vi "sonar_position_difference.vi"(2 "Obstacles":dbl[][](array[numeric]), 3 "Car.lvclass":refnum<class "Car.lvclass">, 4 "Sonar Readings":dbl[](array[numeric])) -> (0 "Y Difference":dbl, 1 "X Difference":dbl)   [LabVIEW 2015]
uses:
  class/Car.lvclass
  class/SonarSensor.lvclass
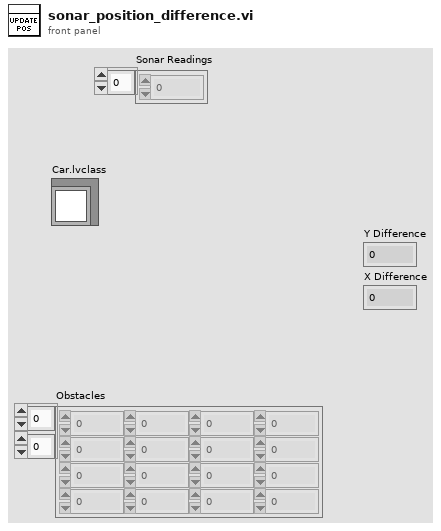
[diagram p1: front panel]
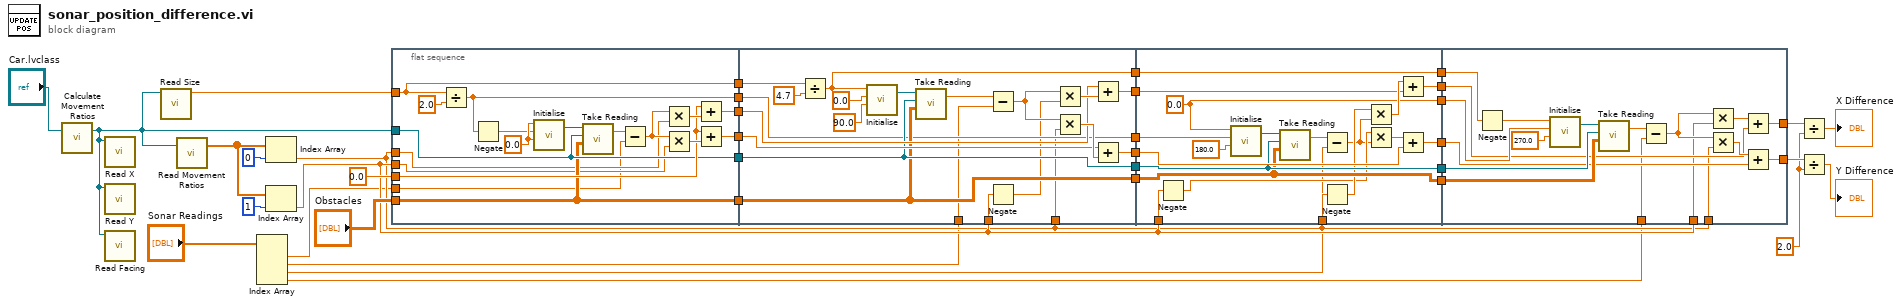
[diagram p0: block diagram]
diagram:
  w11 = 2.0 ("y")
  n1 = call "Calculate Movement Ratios.vi"("Car.lvclass"="Car.lvclass") -> ("Car.lvclass 2"=w1:refnum<class "Car.lvclass">)  [unwired: 1 in, 1 out]
  n2 = call "Read X.vi"("Car.lvclass"=w1) -> ()  [unwired: 9 in, 2 out]
  n3 = call "Read Y.vi"("Car.lvclass"=w1) -> ()  [unwired: 9 in, 2 out]
  n4 = call "Read Facing.vi"("Car.lvclass"=w1) -> ()  [unwired: 9 in, 2 out]
  n5 = call "Read Size.vi"("Car.lvclass"=w1) -> ("Size"=w4:dbl)  [unwired: 9 in, 1 out]
  n6 = call "Read Movement Ratios.vi"("Car.lvclass"=w1) -> ("Array"=w2:dbl[])  [unwired: 1 in, 1 out]
  n7 = Index Array(array="Sonar Readings") -> (element #1=w8:dbl, element #2=w7:dbl, element #3=w6:dbl, element #4=w5:dbl)  [unwired: 4 in]
  n8 = Index Array(array=w2, index=0) -> (element=w15:dbl)
  n9 = Index Array(array=w2, index=1) -> (element=w16:dbl)
  n10 = flat-sequence {
    tunnel: w1 -> [w44]
    tunnel: "Obstacles" -> [w43]
    tunnel: w15 -> [w42]
    tunnel: w16 -> [w41]
    tunnel: 0.0 -> [w48]
    tunnel: [w50] -> w34
    tunnel: [w49] -> w33
    tunnel: w4 -> [w45]
    tunnel: [w45] -> w32
    tunnel: [w44] -> w31
    tunnel: [w43] -> w30
    tunnel: [w40] -> w26
    tunnel: w8 -> [w39]
    tunnel: w34 -> [w69]
    tunnel: w33 -> [w68]
    tunnel: w32 -> [w76]
    tunnel: w31 -> [w67]
    tunnel: w30 -> [w66]
    tunnel: [w67] -> w29
    tunnel: [w66] -> w28
    tunnel: [w65] -> w27
    tunnel: w26 -> [w65]
    tunnel: [w64] -> w25
    tunnel: [w63] -> w24
    tunnel: [w62] -> w20
    tunnel: w15 -> [w61]
    tunnel: w16 -> [w59]
    tunnel: w7 -> [w57]
    tunnel: w29 -> [w89]
    tunnel: w28 -> [w88]
    tunnel: w27 -> [w95]
    tunnel: w25 -> [w91]
    tunnel: w24 -> [w90]
    tunnel: [w89] -> w23
    tunnel: [w88] -> w22
    tunnel: [w87] -> w21
    tunnel: w20 -> [w86]
    tunnel: [w86] -> w19
    tunnel: [w84] -> w18
    tunnel: [w83] -> w17
    tunnel: w15 -> [w82]
    tunnel: w16 -> [w80]
    tunnel: w6 -> [w79]
    tunnel: w23 -> [w114]
    tunnel: w22 -> [w113]
    tunnel: w21 -> [w112]
    tunnel: w19 -> [w110]
    tunnel: w18 -> [w105]
    tunnel: w17 -> [w104]
    tunnel: [w103] -> w12
    tunnel: [w102] -> w13
    tunnel: w16 -> [w101]
    tunnel: w15 -> [w98]
    tunnel: w5 -> [w99]
    frame #0 {
      w56 = 0.0
      n11 = Divide(x=w45, y=2.0) -> (x/y=w40:dbl)
      n12 = Negate(x=w40) -> (-x=w46:dbl)
      n13 = call "Initialise.vi"("Facing"=w56, "Y"=w46, "X"=w56) -> ("SonarSensor.lvclass"=w55:refnum<class "SonarSensor.lvclass">)  [unwired: 1 in, 1 out]
      n14 = call "Take Reading.vi"("Obstacle Boundries"=w43, "Car.lvclass"=w44, "SonarSensor.lvclass"=w55) -> ("Distance Read"=w54:dbl)  [unwired: 1 in, 1 out]
      n15 = Subtract(x=w54, y=w39) -> (x-y=w53:dbl)
      n16 = Multiply(x=w53, y=w42) -> (x*y=w52:dbl)
      n17 = Multiply(x=w53, y=w41) -> (x*y=w51:dbl)
      n18 = Add(x=w48, y=w52) -> (x+y=w49:dbl)
      n19 = Add(x=w48, y=w51) -> (x+y=w50:dbl)
    }
    frame #1 {
      n20 = Divide(x=w76, y=4.7) -> (x/y=w62:dbl)
      n21 = call "Initialise.vi"("Facing"=90.0, "Y"=0.0, "X"=w62) -> ("SonarSensor.lvclass"=w73:refnum<class "SonarSensor.lvclass">)  [unwired: 1 in, 1 out]
      n22 = call "Take Reading.vi"("Obstacle Boundries"=w66, "Car.lvclass"=w67, "SonarSensor.lvclass"=w73) -> ("Distance Read"=w58:dbl)  [unwired: 1 in, 1 out]
      n23 = Subtract(x=w58, y=w57) -> (x-y=w72:dbl)
      n24 = Negate(x=w59) -> (-x=w60:dbl)
      n25 = Multiply(x=w72, y=w60) -> (x*y=w71:dbl)
      n26 = Multiply(x=w72, y=w61) -> (x*y=w70:dbl)
      n27 = Add(x=w68, y=w71) -> (x+y=w63:dbl)
      n28 = Add(x=w69, y=w70) -> (x+y=w64:dbl)
    }
    frame #2 {
      w87 = 0.0 ("X")
      n29 = Negate(x=w80) -> (-x=w81:dbl)
      n30 = call "Initialise.vi"("Facing"=180.0, "Y"=w95, "X"=w87) -> ("SonarSensor.lvclass"=w97:refnum<class "SonarSensor.lvclass">)  [unwired: 1 in, 1 out]
      n31 = call "Take Reading.vi"("Obstacle Boundries"=w88, "Car.lvclass"=w89, "SonarSensor.lvclass"=w97) -> ("Distance Read"=w94:dbl)  [unwired: 1 in, 1 out]
      n32 = Subtract(x=w94, y=w79) -> (x-y=w78:dbl)
      n33 = Negate(x=w82) -> (-x=w85:dbl)
      n34 = Multiply(x=w85, y=w78) -> (x*y=w93:dbl)
      n35 = Multiply(x=w81, y=w78) -> (x*y=w92:dbl)
      n36 = Add(x=w93, y=w90) -> (x+y=w84:dbl)
      n37 = Add(x=w92, y=w91) -> (x+y=w83:dbl)
    }
    frame #3 {
      n38 = Negate(x=w110) -> (-x=w111:dbl)
      n39 = call "Initialise.vi"("Facing"=270.0, "Y"=w112, "X"=w111) -> ("SonarSensor.lvclass"=w115:refnum<class "SonarSensor.lvclass">)  [unwired: 1 in, 1 out]
      n40 = call "Take Reading.vi"("Obstacle Boundries"=w113, "Car.lvclass"=w114, "SonarSensor.lvclass"=w115) -> ("Distance Read"=w100:dbl)  [unwired: 1 in, 1 out]
      n41 = Subtract(x=w100, y=w99) -> (x-y=w108:dbl)
      n42 = Multiply(x=w108, y=w101) -> (x*y=w107:dbl)
      n43 = Multiply(x=w108, y=w98) -> (x*y=w106:dbl)
      n44 = Add(x=w107, y=w105) -> (x+y=w103:dbl)
      n45 = Add(x=w106, y=w104) -> (x+y=w102:dbl)
    }
  }
  n46 = Divide(x=w12, y=w11) -> (x/y=→"X Difference":dbl)
  n47 = Divide(x=w13, y=w11) -> (x/y=→"Y Difference":dbl)
